vi "Relay (DBL).vi"(2 "initialize":bool, 3 "output when on/off":T1={"output when on"=1.0, "output when off"=0.0} {"output when off" format="%.2f"; "output when on" format="%.2f"}, 4 "switch on/off point":T2 {"switch off point" format="%.2f"; "switch on point" format="%.2f"}, 5 "input point":dbl format="%.2f") -> (1 "output point":dbl format="%.2f")   [LabVIEW 2017, in "NI_AdvCtrl_nonlinear.lvlib"]
doc: "LabVIEW no longer supports this VI. You can obtain similar functionality by installing the LabVIEW Simulation Module.\n\nSwitches between two constants. When the relay is on, it remains on until input drops below the value of switch off point. When the relay is off, it remains off until input exceeds the value of switch on point. The relay is predefined in the on state."
uses:
  <vilib>/addons/control/advanced/NI_AdvCtrl_nonlinear.lvlib
  <vilib>/addons/control/advanced/NI_AdvCtrl_continuous linear.lvlib
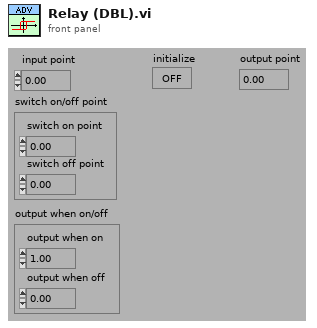
[diagram p1: front panel]
types:
  T1 = cluster{"output when on":dbl, "output when off":dbl}
  T2 = cluster{"switch on point":dbl, "switch off point":dbl}
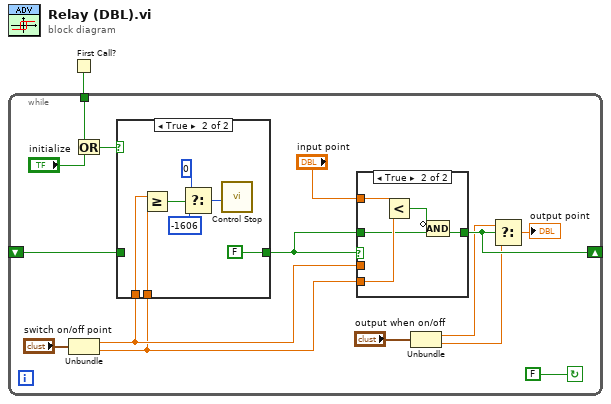
[diagram p0: block diagram]
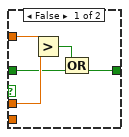
[diagram p3: hidden frame]
diagram:
  n1 = First Call?() -> (First Call?: T/F=w1:bool)
  n2 = while {
    tunnel: w1 -> [w11]
    shift-left: _ -> [w15]
    shift-right: [w8] -> _
    stop <- FALSE continue-if-true
    n3 = Unbundle("switch on/off point") -> ("switch on point"=w6:dbl, "switch off point"=w5:dbl)
    n4 = Or(x=w11, y="initialize") -> (x .or. y?=w12:bool)
    n5 = case shown="True" w12 {
      tunnel: w15 -> [w17 _]
      tunnel: [w17 FALSE] -> w14
      tunnel: w6 -> [_ w23]
      tunnel: w5 -> [_ w22]
      frame False {
      }
      frame True {
        n6 = Greater Or Equal?(x=w23, y=w22) -> (x >= y?=w19:bool)
        n7 = Select(t=0, s=w19, f=-1606) -> (s? t:f=w18:i32)
        n8 = call <vilib>:"Control Stop.vi"("error"=w18) -> ()  [unwired: 2 out]
      }
    }
    n9 = case shown="True" w14 {
      tunnel: "input point" -> [w29 w34]
      tunnel: w5 -> [_ w33]
      tunnel: w14 -> [w26 w31]
      tunnel: [w25 w30] -> w8
      tunnel: w6 -> [w28 _]
      frame False {
        n10 = Greater?(x=w29, y=w28) -> (0:w27:bool)
        n11 = Compound Arithmetic op=OR(w27, w26) -> (w25:bool)
      }
      frame True {
        n12 = Less?(x=w34, y=w33) -> (x < y?=w32:bool)
        n13 = Compound Arithmetic op=AND(invert w32, w31) -> (w30:bool)
      }
    }
    n14 = Unbundle("output when on/off") -> ("output when on"=w2:dbl, "output when off"=w3:dbl)
    n15 = Select(t=w2, s=w8, f=w3) -> (s? t:f=→"output point":dbl)
  }
